vi "sub_SDR_mimo_MuxPorts.vi"(8 "Port 2 in":cdb[](array[numeric]), 11 "Port 1 in":cdb[](array[numeric])) -> (2 "Data out (2D)":cdb[][](array[numeric]))   [LabVIEW 2012]
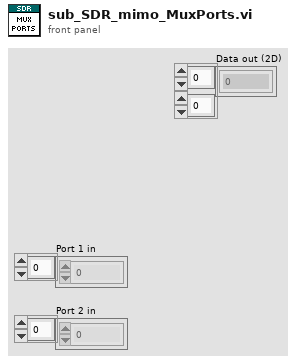
[diagram p1: front panel]
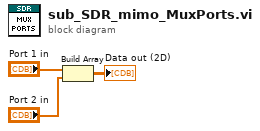
[diagram p0: block diagram]
diagram:
  n1 = Build Array("Port 1 in", "Port 2 in") -> (→"Data out (2D)":cdb[][])
